vi "ObtainQueue.vi"(6 "max queue size (-1, unlimited)":i32=-1, 7 "Queue Name":string, 8 "Error In":errorcluster, 9 "MyPluginsClass":refnum<class "MyPluginsBase.lvclass">, 10 "Message Data":variant, 11 "InitialMessage":string="Initialize") -> (0 "Error Out":errorcluster, 3 "queue out":refnum<queue>)   [LabVIEW 2018, in "MyPluggableModule.lvlib"]
doc: "This creates or recreates the queue name and obtains a reference to the queue."
uses:
  MyPluggableModule.lvlib
  MyPlugins/MyPluginBaseClass/MyPluginsBase.lvclass
  PublicAPI/Arguments/Messages/clMessage.ctl
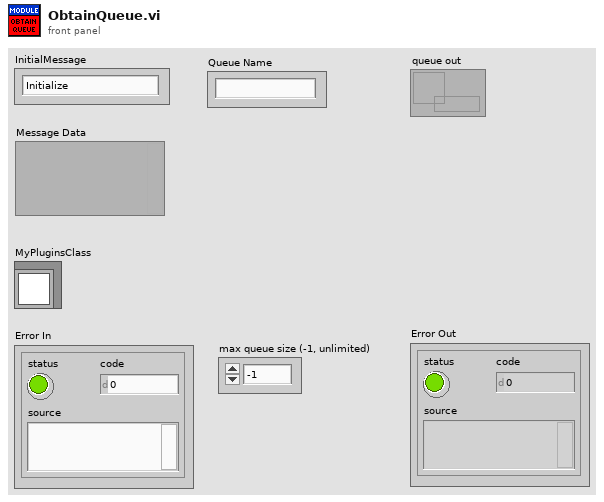
[diagram p1: front panel]
types:
  T1 = typedef "MyPluggableModule.lvlib/clMessage.ctl" = cluster{"Message":string, "Message Data":variant, "MyPluginsClass":refnum<class "MyPluginsBase.lvclass">}
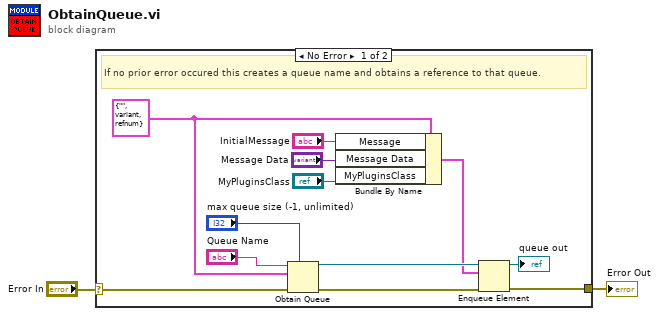
[diagram p0: block diagram]
diagram:
  n1 = case shown="No Error" "Error In" {
    selector: "Error In" -> [w14 w15]
    tunnel: [w9 w15] -> w1
    frame No Error {
      w5 = T1 {"Message"="", "Message Data"=variant, "MyPluginsClass"=refnum} ("clMessage")
      # "If no prior error occured this creates a queue name and obtains a reference to that queue."
      n2 = Obtain Queue(max queue size (-1, unlimited)="max queue size (-1, unlimited)", name (unnamed)="Queue Name", element data type=w5, error in (no error)=w14) -> (queue out=w13:refnum<queue>, error out=w10:errorcluster)  [unwired: 1 in, 1 out]
      n3 = Bundle By Name(cluster=w5, "Message"="InitialMessage", "Message Data"="Message Data", "MyPluginsClass"="MyPluginsClass") -> (w11:T1)
      n4 = Enqueue Element(queue=w13, element=w11, error in (no error)=w10) -> (queue out=→"queue out":refnum<queue>, error out=w9:errorcluster)  [unwired: 1 in, 1 out]
    }
    frame Error {
    }
  }
  "Error Out" <- w1
